vi "Signal Generator Control.vi"(8 "error in":errorcluster, 9 "Waveform Data":T1, 10 "Device":refnum<k15>, 11 "Command":T2) -> (0 "error out":errorcluster, 2 "Device Out":refnum<k15>)   [LabVIEW 2013]
doc: "The VI will control the behavior of a signal generator"
uses:
  Sig Gen Control Command.ctl
  Waveform Details Control.ctl
  Globals/Test Criteria Global.vi
  <instrlib>/niRFSG/niRFSG.llb/niRFSG Write Arb Waveform (I-Q).vi
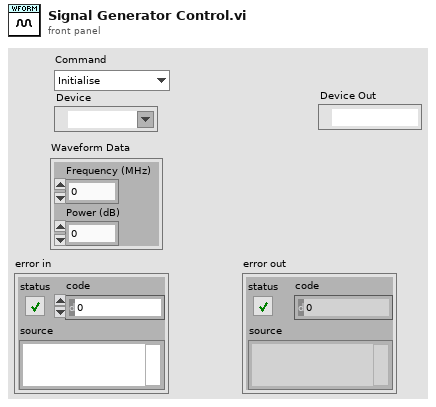
[diagram p1: front panel]
types:
  T1 = typedef "Waveform Details Control.ctl" = cluster{"Power (dB)":dbl, "Frequency (MHz)":u32}
  T2 = typedef "Sig Gen Control Command.ctl" = enum16{"Initialise", "Start", "Stop", "Set Frequency", "Set Power", "Send Packet"}
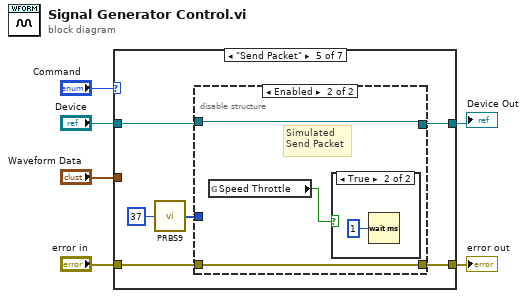
[diagram p0: block diagram]
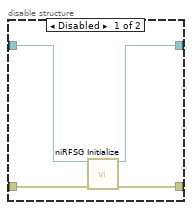
[diagram p3: hidden frame]
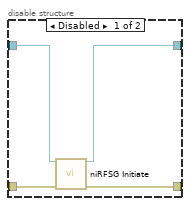
[diagram p6: hidden frame]
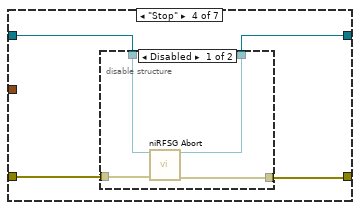
[diagram p7: hidden frame]
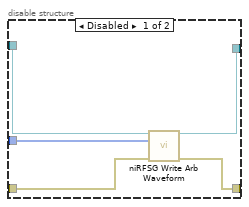
[diagram p9: hidden frame]
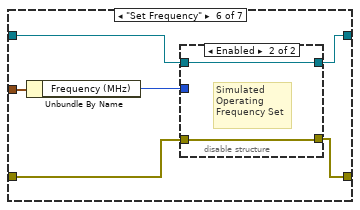
[diagram p11: hidden frame]
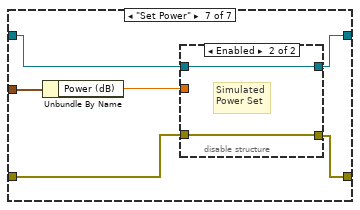
[diagram p13: hidden frame]
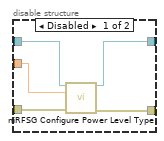
[diagram p14: hidden frame]
diagram:
  n1 = case shown="\"Send Packet\"" "Command" {
    tunnel: "Device" -> [w10 w17 w20 w30 w42 w55 w66]
    tunnel: "error in" -> [w9 w18 w22 w32 w44 w57 w65]
    tunnel: [w8 w18 w21 w31 w43 w56 w64] -> w4
    tunnel: "Waveform Data" -> [_ _ _ _ _ w59 w68]
    tunnel: [w7 w17 w19 w29 w39 w54 w63] -> w1
    frame "Initialise" {
      n2 = disable-structure shown="Enabled" {
        disable-tunnel: w10 -> [w14 w15]
        disable-tunnel: w9 -> [w13 w16]
        disable-tunnel: [w12 w16] -> w8
        disable-tunnel: [w11 w15] -> w7
        frame Disabled {
          n3 = call <instrlib>:"niRFSG Initialize.vi"("resource name"=w14, "error in"=w13) -> ("instrument handle"=w11:refnum<k15>, "error out"=w12:errorcluster)  [unwired: 12 in]
        }
        frame Enabled {
          # "Simulated\nInitialise Step"
        }
      }
    }
    frame Default {
    }
    frame "Start" {
      n4 = disable-structure shown="Enabled" {
        disable-tunnel: w22 -> [w26 w28]
        disable-tunnel: [w25 w28] -> w21
        disable-tunnel: w20 -> [w24 w27]
        disable-tunnel: [w23 w27] -> w19
        frame Disabled {
          n5 = call <instrlib>:"niRFSG Initiate.vi"("instrument handle"=w24, "error in"=w26) -> ("instrument handle out"=w23:refnum<k15>, "error out"=w25:errorcluster)  [unwired: 12 in]
        }
        frame Enabled {
          # "Simulated\n'Start'"
        }
      }
    }
    frame "Stop" {
      n6 = disable-structure shown="Disabled" {
        disable-tunnel: w32 -> [w36 w38]
        disable-tunnel: [w35 w38] -> w31
        disable-tunnel: w30 -> [w34 w37]
        disable-tunnel: [w33 w37] -> w29
        frame Disabled {
          n7 = call <instrlib>:"niRFSG Abort.vi"("instrument handle"=w34, "error in"=w36) -> ("instrument handle out"=w33:refnum<k15>, "error out"=w35:errorcluster)  [unwired: 12 in]
        }
        frame Enabled {
          # "Simulated Stop"
        }
      }
    }
    frame "Send Packet" {
      n8 = call "PRBS9.vi"("Size (Octets)"=37) -> ("Byte Array"=w41:u8[])
      n9 = disable-structure shown="Enabled" {
        disable-tunnel: w44 -> [w49 w52]
        disable-tunnel: [w48 w52] -> w43
        disable-tunnel: w42 -> [w47 w51]
        disable-tunnel: w41 -> [w46 _]
        disable-tunnel: [w45 w51] -> w39
        frame Disabled {
          n10 = call-poly <instrlib>:"niRFSG Write Arb Waveform.vi"("instrument handle"=w47, "I Data"=w46, "error in"=w49) -> ("instrument handle out"=w45:refnum<k15>, "error out"=w48:errorcluster)  [unwired: 11 in]
        }
        frame Enabled {
          # "Simulated\nSend Packet"
          n11 = global read "Test Criteria Global.vi" "Speed Throttle"() -> (w50:bool)
          n12 = case shown="True" w50 {
            frame False {
            }
            frame True {
              n13 = Wait (ms)(milliseconds to wait=u32 1) -> ()  [unwired: 1 out]
            }
          }
        }
      }
    }
    frame "Set Frequency" {
      n14 = Unbundle By Name(w59) -> ("Frequency (MHz)"=w58:u32)
      n15 = disable-structure shown="Enabled" {
        disable-tunnel: w58 -> [_ _]
        disable-tunnel: w57 -> [_ w62]
        disable-tunnel: [_ w62] -> w56
        disable-tunnel: w55 -> [w60 w61]
        disable-tunnel: [w60 w61] -> w54
        frame Disabled {
        }
        frame Enabled {
          # "Simulated\nOperating\nFrequency Set"
        }
      }
    }
    frame "Set Power" {
      n16 = Unbundle By Name(w68) -> ("Power (dB)"=w67:dbl)
      n17 = disable-structure shown="Enabled" {
        disable-tunnel: w67 -> [w70 _]
        disable-tunnel: w66 -> [w71 w74]
        disable-tunnel: w65 -> [w73 w75]
        disable-tunnel: [w72 w75] -> w64
        disable-tunnel: [w69 w74] -> w63
        frame Disabled {
          n18 = call <instrlib>:"niRFSG Configure Power Level Type.vi"("instrument handle"=w71, "power level type"=w70, "error in"=w73) -> ("instrument handle out"=w69:refnum<k15>, "error out"=w72:errorcluster)  [unwired: 11 in]
        }
        frame Enabled {
          # "Simulated\nPower Set"
        }
      }
    }
  }
  "error out" <- w4
  "Device Out" <- w1
